vi "Add TF to Project.vi"   [LabVIEW 2020]
uses:
  Framework/Process/Process.lvclass
types:
  T1 = enum32{"Invalid", "Standard", "Closed", "Hidden", "Minimized", "Maximized"}
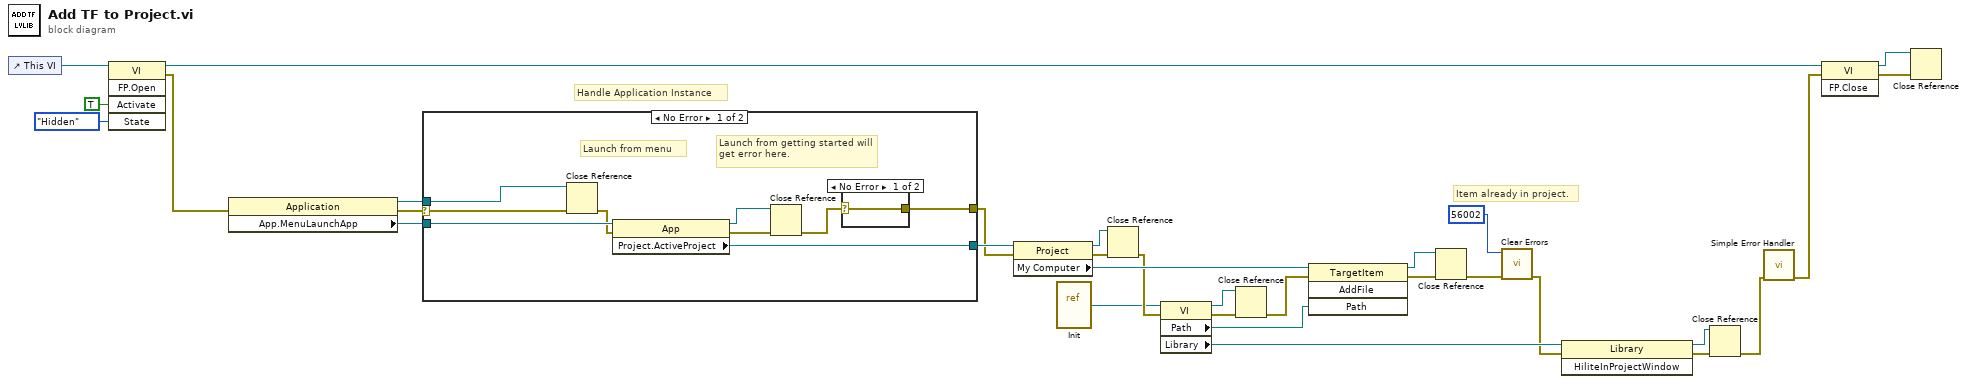
[diagram p0: block diagram]
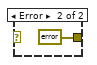
[diagram p2: hidden frame]
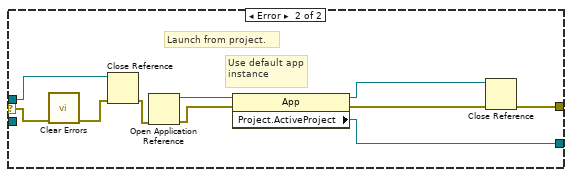
[diagram p3: hidden frame]
diagram:
  # "Item already in project."
  # "Handle Application Instance"
  n1 = control-ref of="This VI"() -> (w3:refnum<vi>)
  n2 = invoke class="VI" method="FP.Open"(reference=w3, "Activate"=TRUE ("Activate?"), "State"=T1."Hidden") -> (reference out=w1:refnum<vi>, error out=w2:errorcluster)  [unwired: 2 in, 3 out]
  n3 = property class="Application"(error in=w2) -> (reference out=w29:refnum<vi>, error out=w30:errorcluster, "App.MenuLaunchApp"=w31:refnum<vi>)  [unwired: 1 in]
  n4 = case shown="No Error" w30 {
    selector: w30 -> [w39 w50]
    tunnel: w31 -> [w38 _]
    tunnel: w29 -> [w40 w49]
    tunnel: [w34 w46] -> w28
    tunnel: [w32 w44] -> w27
    frame No Error {
      # "Launch from getting started will get error here."
      # "Launch from menu"
      n5 = Close Reference(reference=w40, error in (no error)=w39) -> (error out=w37:errorcluster)
      n6 = property class="App"(reference=w38, error in=w37) -> (reference out=w36:refnum<vi>, error out=w35:errorcluster, "Project.ActiveProject"=w34:refnum<vi>)
      n7 = Close Reference(reference=w36, error in (no error)=w35) -> (error out=w33:errorcluster)
      n8 = case shown="No Error" w33 {
        selector: w33 -> [w41 _]
        tunnel: [w41 errorcluster {"status"=TRUE, "code"=42, "source"="Quick Launch can only be enabled from within a LabVIEW Project. "} ("error constant")] -> w32
        frame No Error {
        }
        frame Error {
        }
      }
    }
    frame Error {
      # "Launch from project."
      # "Use default app instance"
      n9 = call <vilib>:"Clear Errors.vi"("error in (no error)"=w50) -> ("error out"=w48:errorcluster)  [unwired: 5 in, 1 out]
      n10 = Close Reference(reference=w49, error in (no error)=w48) -> (error out=w47:errorcluster)
      n11 = Open Application Reference(8:w47) -> (0:w51:errorcluster, 3:w52:refnum<vi>)  [unwired: 3 in]
      n12 = property class="App"(reference=w52, error in=w51) -> (reference out=w43:refnum<vi>, error out=w45:errorcluster, "Project.ActiveProject"=w46:refnum<vi>)
      n13 = Close Reference(reference=w43, error in (no error)=w45) -> (error out=w44:errorcluster)
    }
  }
  n14 = property class="Project"(reference=w28, error in=w27) -> (reference out=w25:refnum<vi>, error out=w24:errorcluster, "My Computer"=w26:refnum<vi>)
  n15 = vi-ref "Init.vi"() -> (w9:refnum<vi>)
  n16 = Close Reference(reference=w25, error in (no error)=w24) -> (error out=w18:errorcluster)
  n17 = property class="VI"(reference=w9, error in=w18) -> (reference out=w19:refnum<vi>, error out=w20:errorcluster, "Path"=w21:path, "Library"=w14:refnum<vi>)
  n18 = Close Reference(reference=w19, error in (no error)=w20) -> (error out=w17:errorcluster)
  n19 = invoke class="TargetItem" method="AddFile"(reference=w26, error in=w17, "Path"=w21) -> (reference out=w22:refnum<vi>, error out=w23:errorcluster)  [unwired: 1 in, 2 out]
  n20 = Close Reference(reference=w22, error in (no error)=w23) -> (error out=w16:errorcluster)
  n21 = call <vilib>:"Clear Errors.vi"("error in (no error)"=w16, "specific error code to clear (0: all)"=56002) -> ("error out"=w11:errorcluster)  [unwired: 4 in, 1 out]
  n22 = invoke class="Library" method="HiliteInProjectWindow"(reference=w14, error in=w11) -> (reference out=w12:refnum<vi>, error out=w13:errorcluster)  [unwired: 1 in, 1 out]
  n23 = Close Reference(reference=w12, error in (no error)=w13) -> (error out=w10:errorcluster)
  n24 = call <vilib>:"Simple Error Handler.vi"("error in (no error)"=w10) -> ("error out"=w8:errorcluster)  [unwired: 4 in, 4 out]
  n25 = invoke class="VI" method="FP.Close"(reference=w1, error in=w8) -> (reference out=w7:refnum<vi>, error out=w6:errorcluster)  [unwired: 1 in, 1 out]
  n26 = Close Reference(reference=w7, error in (no error)=w6) -> ()  [unwired: 1 out]
